vi "Get.vi"(11 "Integer in":refnum<class "Integer.lvclass">) -> (2 "Value":i64)   [LabVIEW 2022 SP3, in "Conditum.lvlib" / "Columns.lvlib" / "Integer.lvclass"]
uses:
  Integer.lvclass
  Integer.lvclass/Integer.ctl
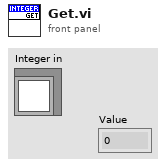
[diagram p1: front panel]
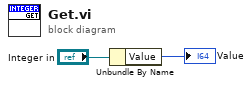
[diagram p0: block diagram]
diagram:
  n1 = Unbundle By Name("Integer in") -> ("Value"=→"Value":i64)
